vi "CalcTorque.vi"(8 "error in (no error)":errorcluster, 11 "CAlexData2 in":refnum<class "CAlex2_Data.lvclass">) -> (0 "error out":errorcluster, 1 "Joint Torque Actual":dbl[][](array[numeric]), 2 "Joint Torque Desired":dbl[][](array[numeric]), 3 "CAlexData2 out":refnum<class "CAlex2_Data.lvclass">, 4 "Tension Actual":dbl[][](array[numeric]), 6 "Tension Desired":dbl[][](array[numeric]))   [LabVIEW 2015, in "CAlex2_Data.lvclass"]
uses:
  CAlex2_Data.lvclass
  CAlex2_Data.lvclass/CAlex2_Data.ctl
  Classes/CAlex2/CAlex2.lvclass
  ExpData/ExpData.lvclass
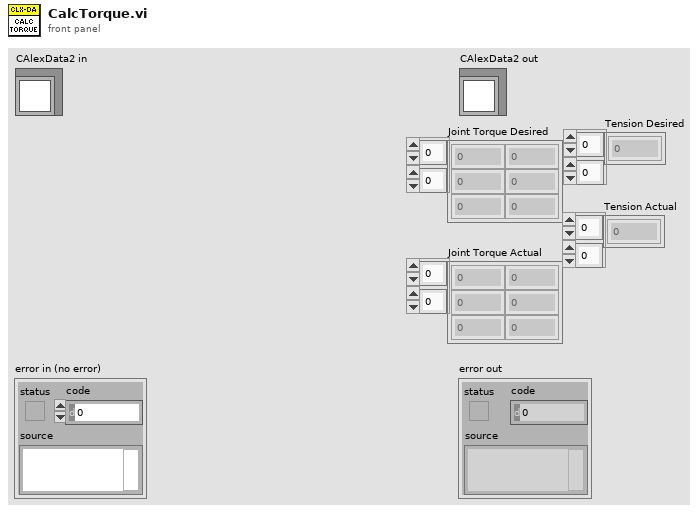
[diagram p1: front panel]
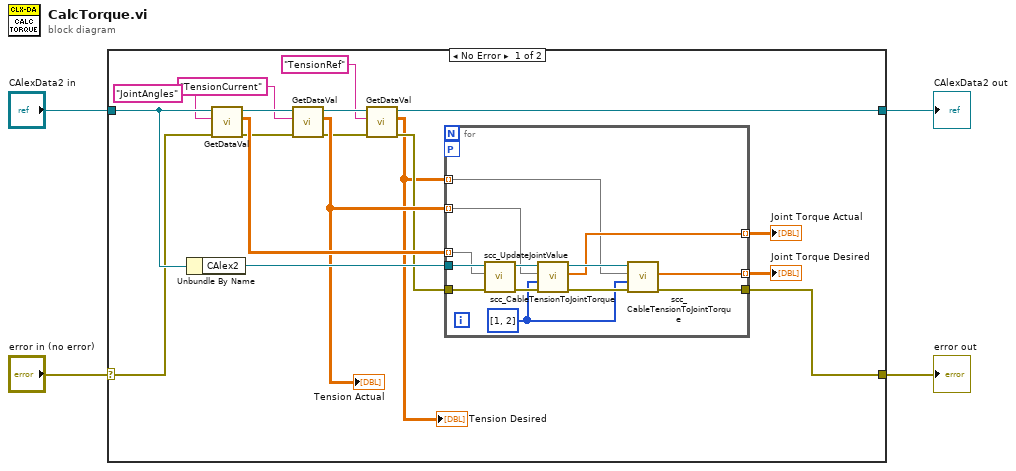
[diagram p0: block diagram]
diagram:
  n1 = case shown="No Error" "error in (no error)" {
    selector: "error in (no error)" -> [w13 w37]
    tunnel: [w12 w37] -> w3
    tunnel: [w9 w36] -> w1
    tunnel: "CAlexData2 in" -> [w21 w36]
    frame No Error {
      n2 = Unbundle By Name(w21) -> ("CAlex2"=w20:refnum<class "CAlex2.lvclass">)
      n3 = call "GetDataVal.vi"("error in (no error)"=w13, "Name"="JointAngles", "CarexMData in"=w21) -> ("error out"=w14:errorcluster, "Data"=w17:dbl[][], "CarexMData out"=w22:refnum<class "CAlex2_Data.lvclass">)  [unwired: 5 in, 1 out]
      n4 = call "GetDataVal.vi"("error in (no error)"=w14, "Name"="TensionCurrent", "CarexMData in"=w22) -> ("error out"=w8:errorcluster, "Data"=w16:dbl[][], "CarexMData out"=w10:refnum<class "CAlex2_Data.lvclass">)  [unwired: 5 in, 1 out]
      "Tension Actual" <- w16
      n5 = call "GetDataVal.vi"("error in (no error)"=w8, "Name"="TensionRef", "CarexMData in"=w10) -> ("error out"=w7:errorcluster, "Data"=w6:dbl[][], "CarexMData out"=w9:refnum<class "CAlex2_Data.lvclass">)  [unwired: 5 in, 1 out]
      "Tension Desired" <- w6
      n6 = for {
        tunnel: w17 -> [w34] mode=indexing
        tunnel: w16 -> [w24] mode=indexing
        tunnel: [w27] -> w15 mode=indexing
        tunnel: w20 -> [w35]
        tunnel: w7 -> [w31]
        tunnel: [w28] -> w12
        workers-P: _ -> [_]
        tunnel: [w26] -> w11 mode=indexing
        tunnel: w6 -> [w23] mode=indexing
        w25 = i32[] [1, 2] ("Locked Joints")
        n7 = call-dynamic "scc_UpdateJointValue.vi"("error in (no error)"=w31, "JointValue (rad|m)"=w34, "C-Alex in"=w35) -> ("error out"=w32:errorcluster, "C-Alex out"=w33:refnum<class "CAlex2.lvclass">)  [unwired: 7 in]
        n8 = call-dynamic "scc_CableTensionToJointTorque.vi"("error in (no error)"=w32, "Locked Joints"=w25, "Cable Tensions"=w24, "SerialChain_Cable in"=w33) -> ("error out"=w29:errorcluster, "Joint Torque"=w26:dbl[], "SerialChain_Cable out"=w30:refnum<class "CAlex2.lvclass">)  [unwired: 5 in]
        n9 = call-dynamic "scc_CableTensionToJointTorque.vi"("error in (no error)"=w29, "Locked Joints"=w25, "Cable Tensions"=w23, "SerialChain_Cable in"=w30) -> ("error out"=w28:errorcluster, "Joint Torque"=w27:dbl[])  [unwired: 5 in, 1 out]
      }
      "Joint Torque Desired" <- w15
      "Joint Torque Actual" <- w11
    }
    frame Error {
    }
  }
  "error out" <- w3
  "CAlexData2 out" <- w1
